vi "Overlay test.vi"() -> ()   [LabVIEW 2015]
panel:
  in  "File Path 2":path=path "C:/Documents and Settings/pursley/Desktop/Images/3229.796.png"
  in  "File Path":path=path "C:/Documents and Settings/pursley/Desktop/Images/result.png"
  out "Overlayed Image":T1(plugin-control)
  out "Grayscale Image":T1(plugin-control)
  out "Color Image":T1(plugin-control)
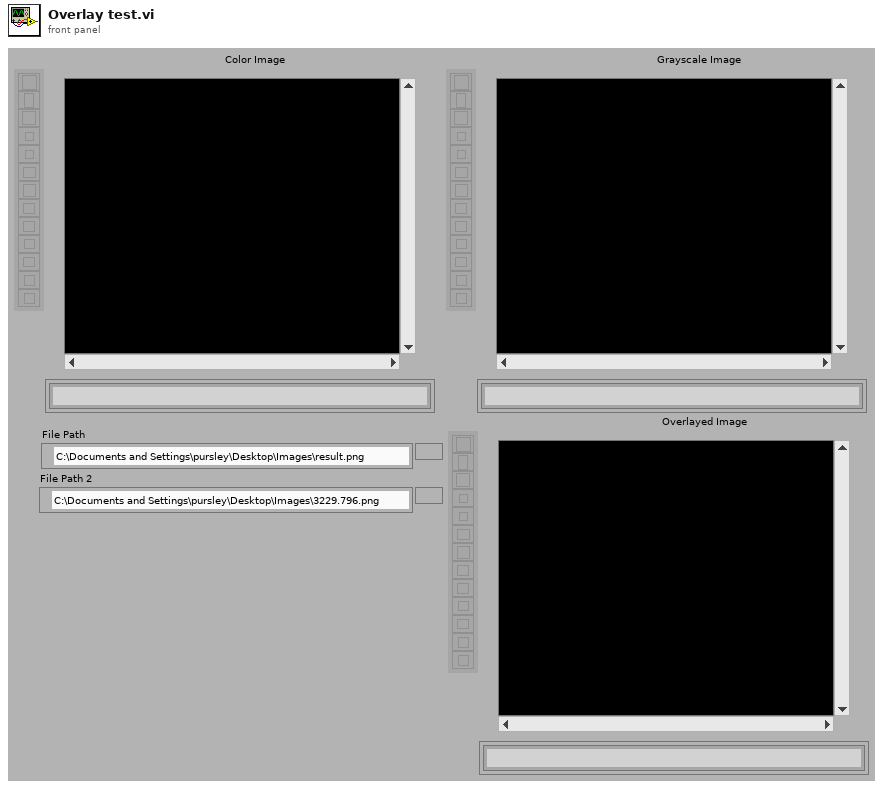
[diagram p1: front panel]
types:
  T1 = typedef "IMAQ Image.ctl" = refnum<image>
  T2 = typedef "Image Type" = u32
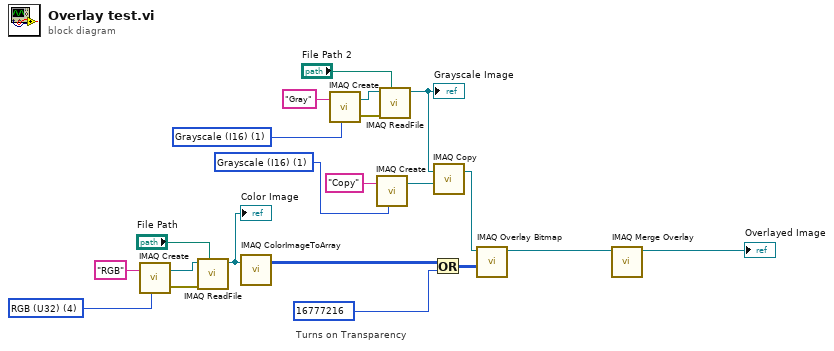
[diagram p0: block diagram]
diagram:
  w8 = T2 1 items=["Grayscale (U8)", "Grayscale (I16)", "Grayscale (SGL)", "Complex (CSG)", "RGB (U32)", "HSL (U32)", "RGB (U64)", "Grayscale (U16)"] ("Image Type")
  w12 = T2 1 items=["Grayscale (U8)", "Grayscale (I16)", "Grayscale (SGL)", "Complex (CSG)", "RGB (U32)", "HSL (U32)", "RGB (U64)", "Grayscale (U16)"] ("Image Type")
  w21 = T2 4 items=["Grayscale (U8)", "Grayscale (I16)", "Grayscale (SGL)", "Complex (CSG)", "RGB (U32)", "HSL (U32)", "RGB (U64)", "Grayscale (U16)"] ("Image Type")
  # "Turns on Transparency"
  n1 = call "IMAQ Create"("Image Name"="RGB", "Image Type"=w21) -> ("New Image"=w18:T1, "error out"=w19:errorcluster)  [unwired: 2 in, 1 out]
  n2 = call "IMAQ ReadFile"("File Path"="File Path", "error in (no error)"=w19, "Image"=w18) -> ("Image Out"=w11:T1)  [unwired: 2 in, 6 out]
  "Color Image" <- w11
  n3 = call "IMAQ ColorImageToArray"("Image"=w11) -> ("Image Pixels (U32)"=w3:u32[][])  [unwired: 2 in, 3 out]
  n4 = call "IMAQ Create"("Image Name"="Gray", "Image Type"=w12) -> ("New Image"=w15:T1, "error out"=w14:errorcluster)  [unwired: 2 in, 1 out]
  n5 = call "IMAQ Create"("Image Name"="Copy", "Image Type"=w8) -> ("New Image"=w6:T1)  [unwired: 2 in, 2 out]
  n6 = call "IMAQ ReadFile"("File Path"="File Path 2", "error in (no error)"=w14, "Image"=w15) -> ("Image Out"=w5:T1)  [unwired: 2 in, 6 out]
  "Grayscale Image" <- w5
  n7 = Or(x=w3, y=u32 16777216 ("Numeric")) -> (x .or. y?=w10:u32[][])
  n8 = call "IMAQ Copy"("Image Dst"=w6, "Image Src"=w5) -> ("Image Dst Out"=w4:T1)  [unwired: 1 in, 4 out]
  n9 = call "IMAQ Overlay Bitmap"("Bitmap"=w10, "Image"=w4) -> ("Image Out"=w1:T1)  [unwired: 3 in, 6 out]
  n10 = call "IMAQ Merge Overlay"("Image Src"=w1) -> ("Image Dst Out"=→"Overlayed Image":T1)  [unwired: 4 in, 6 out]
